vi "Init.vi"(4 "Custom":string[](array[string]), 6 "Concatenate\\Build [T, Concatenate]":bool=TRUE, 8 "error in (no error)":errorcluster, 10 "Data [name]":T1[](array[typedef])=[enum."name"]) -> (0 "error out":errorcluster, 3 "Find First Query out":refnum<class "Add Results Query.lvclass">)   [LabVIEW 2013, in "Add Results Query.lvclass"]
doc: "Copyright 2018, Carya Automatisering, Wiebe Walstra."
uses:
  Add Results Query.lvclass
  Data.ctl
  Add Results Query.lvclass/Add Results Query.ctl
  CConfig Object.lvclass
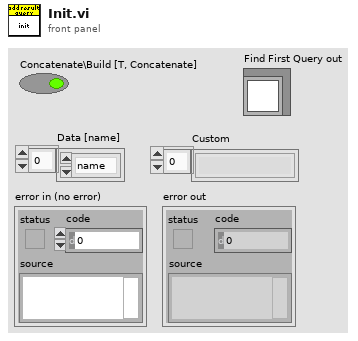
[diagram p1: front panel]
types:
  T1 = typedef "CConfig Object.lvclass/Data.ctl" = enum16{"pre", "name", "middle", "value", "post", "newline", "persistant", "tagged", "type"}
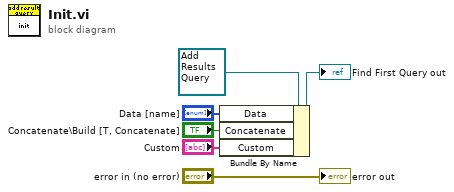
[diagram p0: block diagram]
diagram:
  n1 = Bundle By Name(cluster=refnum<class "Add Results Query.lvclass"> refnum ("Find First Query in"), "Data"="Data [name]", "Concatenate"="Concatenate\\Build [T, Concatenate]", "Custom"="Custom") -> (→"Find First Query out":refnum<class "Add Results Query.lvclass">)
  "error out" <- "error in (no error)"
